vi "snprintf.vi"(7 "para3":u64, 8 "error in (no error)":errorcluster, 9 "para2":string, 10 "para1":string, 11 "para0":i32) -> (0 "error out":errorcluster, 2 "para1 out":string, 3 "function return":string)   [LabVIEW 2020, in "sqlite3.lvlib"]
uses:
  sqlite3.lvlib
  errstr.vi
  bin/sqlite3_64.dll
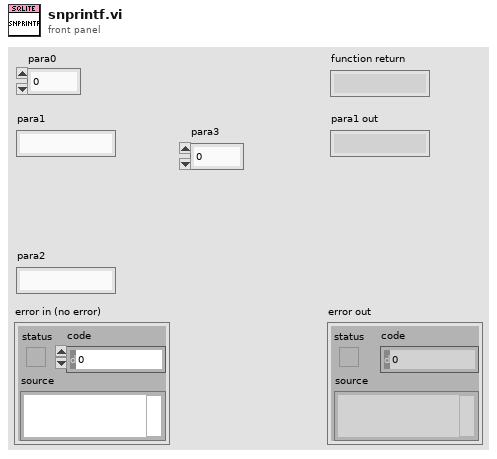
[diagram p1: front panel]
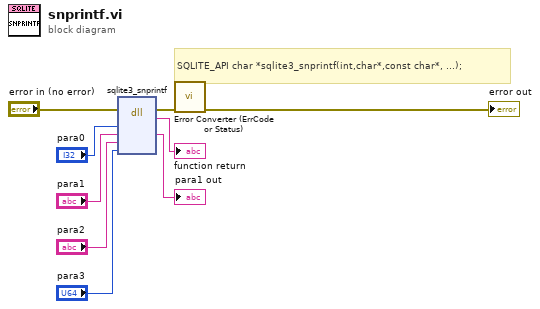
[diagram p0: block diagram]
diagram:
  # "SQLITE_API char *sqlite3_snprintf(int,char*,const char*, ...);"
  n1 = dll-call lib="D:/Project/Labview-Projects/database-configuration/externals/sqlite3/Source/bin/sqlite3_*.*" fn="sqlite3_snprintf"(error in="error in (no error)", "para0"="para0", "para1"="para1", "para2"="para2", "para3"="para3") -> (error out=w2:errorcluster, →"function return":string, "para1"=→"para1 out":string)  [unwired: 5 in, 1 out]
  n2 = call "Error Converter (ErrCode or Status).vi"("error in (no error)"=w2) -> ("error out"=→"error out":errorcluster)  [unwired: 10 in]
